vi "dump data from VIs.vi"(7 "vipb base":path, 8 "error in (no error)":errorcluster, 9 "palette sections":T1(array[cluster]), 10 "assets":path, 11 "docs folder":path) -> (0 "error out":errorcluster)   [LabVIEW 2020]
uses:
  <vilib>/JDP Science/JSONtext/LVClass Serializer/JSONtext LVClass Serializer.lvclass
  sphinx terminal direction.ctl
  sphinx terminal data.ctl
  sphinx item data.ctl
  <vilib>/Utility/Data Type/NI_Data Type.lvlib
  41f7d256-710a-436a-832c-a9b2a359d6cb.vi
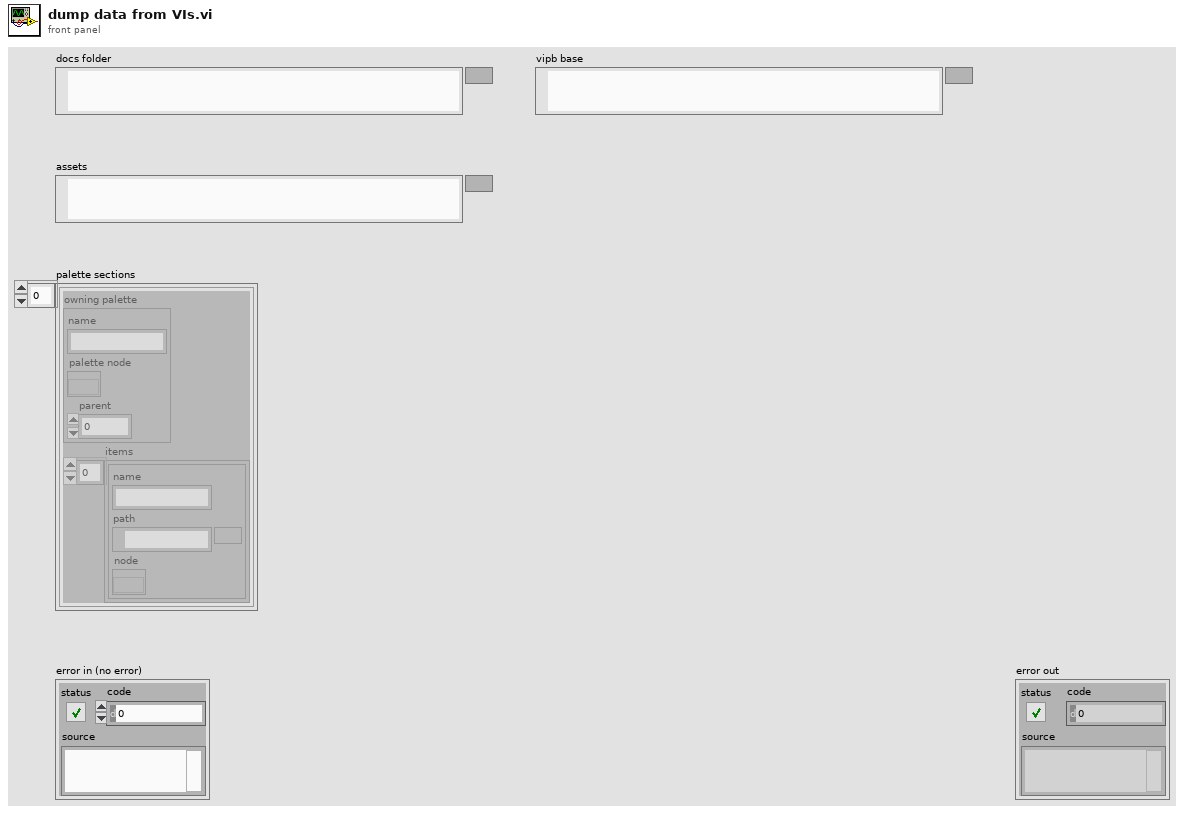
[diagram p1: front panel]
types:
  T1 = cluster{"owning palette":cluster{"name":string, "palette node":refnum<k20>, "parent":i32}, "items":cluster{"name":string, "path":path, "node":refnum<k20>}[]}[]
  T2 = typedef "sphinx item data.ctl" = cluster{"id":string, "kind":string, "path":path, "owner":string, "description":string, "icon":path, "terminals":T3[], "relative palette location":string, "connpane":path, "parent ID":string}
  T3 = typedef "sphinx terminal data.ctl" = cluster{"label":string, "direction":T4, "type":string, "type_id":string, "default":string, "description":string, "tip strip":string, "wiring rule":enum16{"Invalid Wire Rule", "Required", "Recommended", "Optional", "Dynamic Dispatch"}, "caption":string}
  T4 = typedef "sphinx terminal direction.ctl" = enum16{"input", "output"}
  T5 = enum16{"open", "replace", "create", "open or create", "replace or create", "replace or create with confirmation"}
  T6 = cluster{"name":string, "palette node":refnum<k20>, "parent":i32}
  T7 = cluster{"name":string, "path":path, "node":refnum<k20>}[]
  T8 = enum32{"invalid VI type", "Standard VI", "Control VI", "Global VI", "Polymorphic VI", "Configuration VI", "SubSystem", "Facade VI", "Method VI", "Statechart Diagram VI"}
  T9 = cluster{"VIPath":path, "Menu Name":string, "Selector Name":string}[]
  T10 = enum16{"Invalid Wire Rule", "Required", "Recommended", "Optional", "Dynamic Dispatch"}
  T11 = typedef "NI_Data Type.lvlib/Data Type.ctl" = enum8{"Invalid Type", "Void", "I8", "I16", "I32", "I64", "U8", "U16", "U32", "U64", "Single Float", "Double Float", "Extended Float", "Single Complex", "Double Complex", "Extended Complex", "Enum U8", "Enum U16", "Enum U32", "Enum U64", "Single Float With Unit", "Double Float With Unit", "Extended Float With Unit", "Single Complex with Unit", "Double Complex with Unit", "Extended Complex with Unit", "Boolean", "String", "Path", "Picture", "Tag", "Array", "Cluster", "Variant", "LV Variant", "Waveform", "Timestamp", "Digital Waveform", "Digital Data", "ExpressData", "Refnum", "External Data", "VI", "Poly VI", "LabVIEW Class Instance", "Fixed Point", "Set Collection", "Map Collection"}
  T12 = typedef "NI_Data Type.lvlib/Type Definition Info.ctl" = cluster{"Name":string, "Timestamp":u32}
  T13 = typedef "imagedata.ctl" = cluster{"image type":i32, "image depth":i32, "image":u8[], "mask":u8[], "colors":u32[], "Rectangle":cluster{"left":i16, "top":i16, "right":i16, "bottom":i16}}
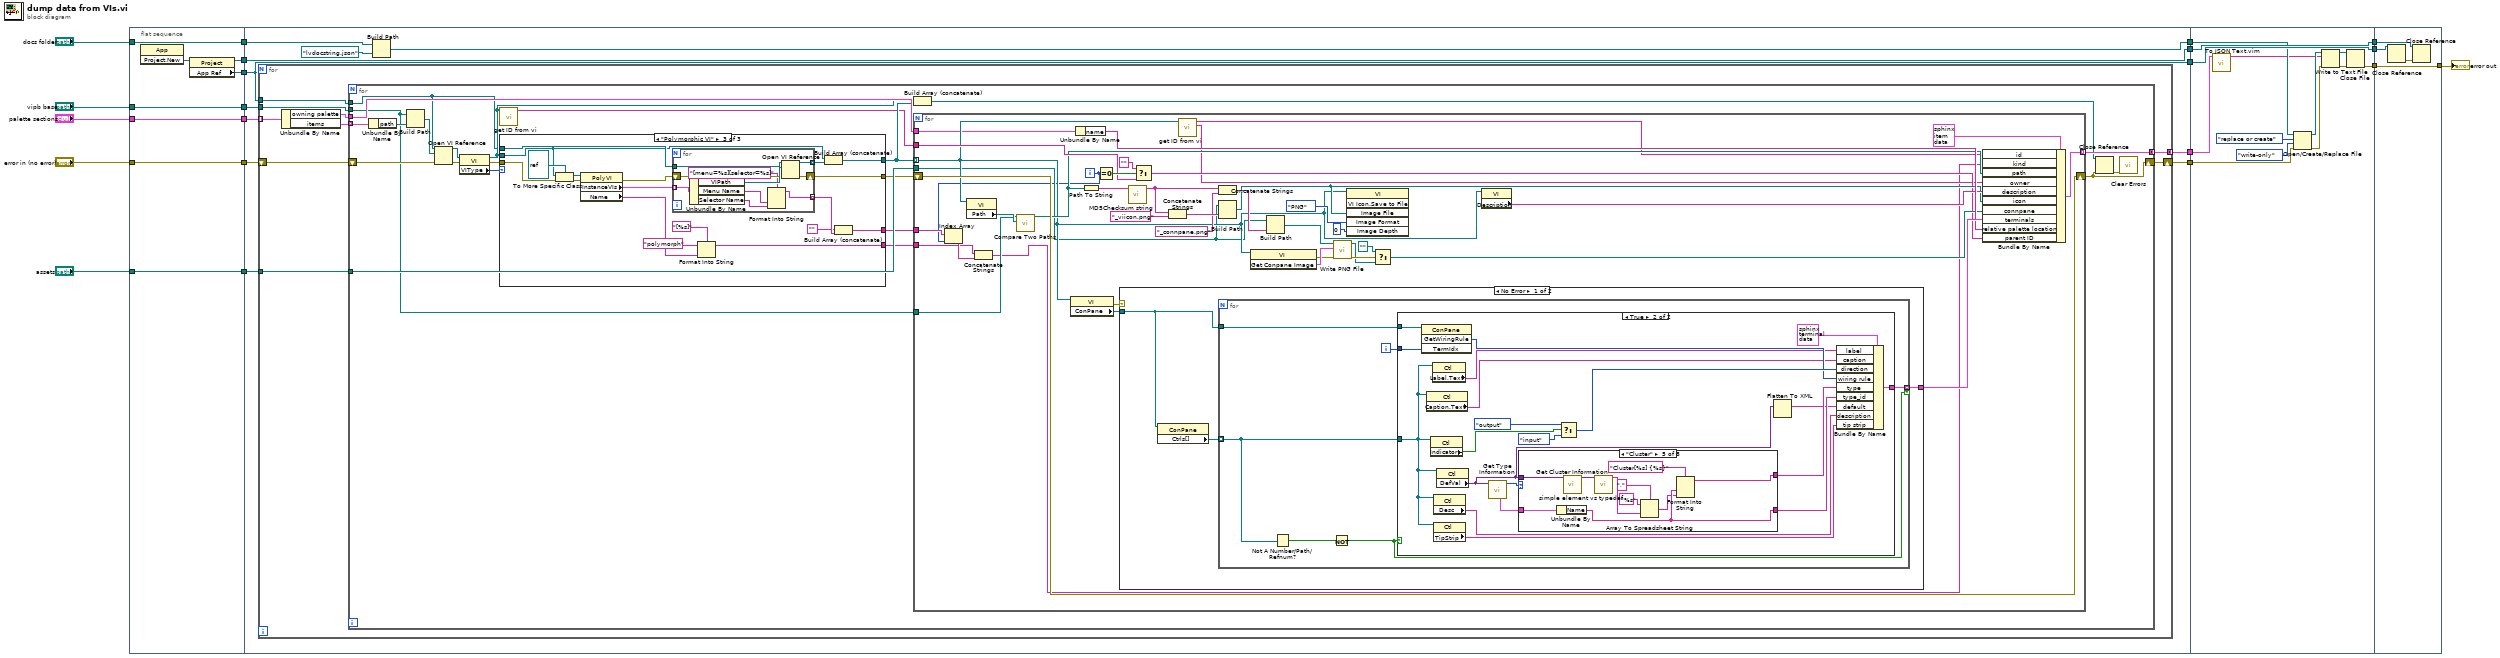
[diagram p0: block diagram]
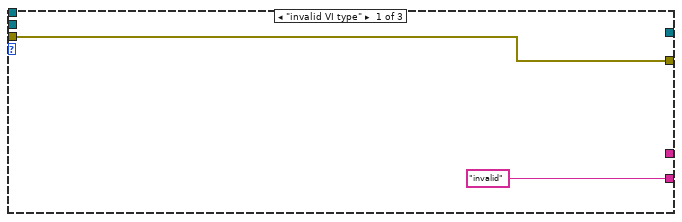
[diagram p2: hidden frame]
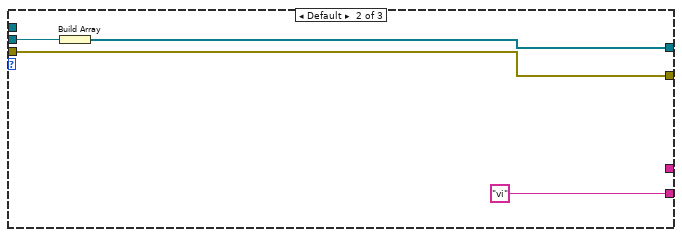
[diagram p3: hidden frame]
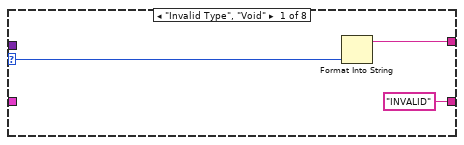
[diagram p5: hidden frame]
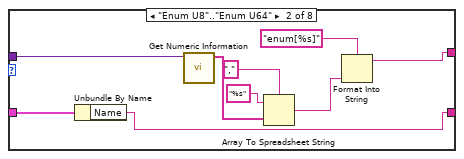
[diagram p6: hidden frame]
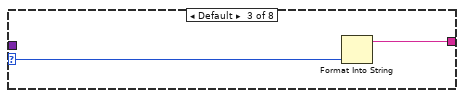
[diagram p7: hidden frame]
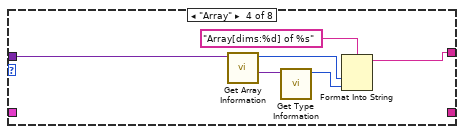
[diagram p8: hidden frame]
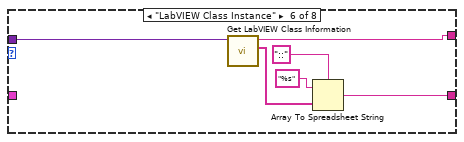
[diagram p9: hidden frame]
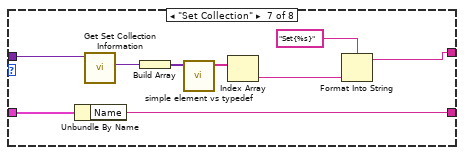
[diagram p10: hidden frame]
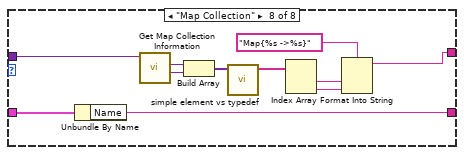
[diagram p11: hidden frame]
diagram:
  n1 = flat-sequence {
    tunnel: "palette sections" -> [w29]
    tunnel: [w29] -> w21
    tunnel: [w27] -> w20
    tunnel: [w26] -> w19
    tunnel: "error in (no error)" -> [w23]
    tunnel: "assets" -> [w25]
    tunnel: [w25] -> w18
    tunnel: [w24] -> w17
    tunnel: "docs folder" -> [w24]
    tunnel: [w23] -> w11
    tunnel: "vipb base" -> [w22]
    tunnel: [w22] -> w9
    tunnel: w21 -> [w40]
    tunnel: w20 -> [w39]
    tunnel: [w39] -> w8
    tunnel: [w38] -> w6
    tunnel: w19 -> [w38]
    tunnel: w18 -> [w37]
    tunnel: w17 -> [w36]
    tunnel: w11 -> [w34]
    tunnel: w9 -> [w33]
    tunnel: [w32] -> w3
    tunnel: [w31] -> w2
    tunnel: [w30] -> w1
    tunnel: w8 -> [w244]
    tunnel: [w244] -> w7
    tunnel: w6 -> [w243]
    tunnel: [w243] -> w5
    tunnel: [w234] -> w4
    tunnel: w3 -> [w238]
    tunnel: w2 -> [w235]
    tunnel: w1 -> [w233]
    tunnel: w7 -> [w247]
    tunnel: w5 -> [w246]
    tunnel: [w245] -> w16
    tunnel: w4 -> [w245]
    frame #0 {
      n2 = invoke class="App" method="Project.New"() -> ("Project:New"=w28:refnum<vi>)  [unwired: 3 in, 2 out]
      n3 = property class="Project"(reference=w28) -> (reference out=w27:refnum<vi>, "App Ref"=w26:refnum<vi>)  [unwired: 1 in, 1 out]
    }
    frame #1 {
      n4 = for {
        tunnel: w40 -> [w49] mode=indexing
        tunnel: w38 -> [w47]
        tunnel: [w45] -> w30 mode=concatenating
        tunnel: w37 -> [w44]
        shift-right: [w42] -> w32
        shift-left: w34 -> [w43]
        tunnel: w33 -> [w41]
        n5 = Unbundle By Name(w49) -> ("owning palette"=w46:T6, "items"=w48:T7)
        n6 = for {
          tunnel: w48 -> [w71] mode=indexing
          tunnel: w47 -> [w54]
          tunnel: w46 -> [w69]
          tunnel: [w68] -> w45 mode=concatenating
          tunnel: w44 -> [w67]
          shift-right: [w58] -> w42
          shift-left: w43 -> [w66]
          tunnel: w41 -> [w51]
          n7 = Unbundle By Name(w71) -> ("path"=w65:path)
          n8 = Build Path(base path=w51, name or relative path=w65) -> (appended path=w64:path)
          n9 = Open VI Reference(application reference (local)=w54, vi path=w64, error in (no error)=w66) -> (vi reference=w62:refnum<vi>, error out=w70:errorcluster)  [unwired: 3 in]
          n10 = property class="VI"(reference=w62, error in=w70) -> (reference out=w59:refnum<vi>, error out=w56:errorcluster, "VIType"=w60:T8)
          n11 = call "get ID from vi.vi"("VI in"=w59) -> ("VI ID"=w52:string)  [unwired: 9 in, 1 out]
          n12 = case shown="\"Polymorphic VI\"" w60 {
            tunnel: w59 -> [_ w77 w82]
            tunnel: [_ w76 w83] -> w61
            tunnel: [w73 w75 w89] -> w57
            tunnel: w56 -> [w73 w75 w95]
            tunnel: ["invalid" ("kind") "vi" ("kind") w81] -> w55
            tunnel: w54 -> [_ _ w91]
            tunnel: [_ _ w79] -> w50
            frame "invalid VI type" {
            }
            frame Default {
              n13 = Build Array(w77) -> (w76:refnum<vi>[])
            }
            frame "Polymorphic VI" {
              n14 = To More Specific Class(target class=refnum<vi> refnum, reference=w82, error in=w95) -> (specific class reference=w86:refnum<vi>, error out=w93:errorcluster)
              n15 = property class="PolyVI"(reference=w86, error in=w93) -> (error out=w90:errorcluster, "InstanceVIs"=w92:T9, "Name"=w85:string)  [unwired: 1 out]
              n16 = for {
                tunnel: w92 -> [w105] mode=indexing
                tunnel: w91 -> [w103]
                shift-right: [w101] -> w89
                shift-left: w90 -> [w102]
                tunnel: [w100] -> w88 mode=indexing
                tunnel: [w97] -> w80 mode=indexing
                n17 = Unbundle By Name(w105) -> ("VIPath"=w104:path, "Menu Name"=w99:string, "Selector Name"=w98:string)
                n18 = Format Into String(format string="[menu=%s][selector=%s]", w99, w98) -> (resulting string=w97:string)  [unwired: 2 in, 1 out]
                n19 = Open VI Reference(application reference (local)=w103, vi path=w104, error in (no error)=w102) -> (vi reference=w100:refnum<vi>, error out=w101:errorcluster)  [unwired: 3 in]
              }
              n20 = Format Into String(format string="[%s]", initial string="polymorph" ("kind"), w85) -> (resulting string=w81:string)  [unwired: 1 in, 1 out]
              n21 = Build Array (concatenate)(w82, w88) -> (w83:refnum<vi>[])
              n22 = Build Array (concatenate)("", w80) -> (w79:string[])
            }
          }
          n23 = Build Array (concatenate)(w59, w61) -> (w63:refnum<vi>[])
          n24 = for {
            tunnel: w69 -> [w112]
            tunnel: [w146] -> w68 mode=indexing
            tunnel: w67 -> [w111]
            shift-right: [w145] -> w58
            shift-left: w57 -> [w145]
            tunnel: w61 -> [w115] mode=indexing
            tunnel: w55 -> [w106]
            tunnel: w52 -> [w119]
            tunnel: w51 -> [w117]
            tunnel: w50 -> [w110]
            i -> [w109]
            n25 = Index Array(array=w110, index=w109) -> (element=w108:string)
            n26 = property class="VI"(reference=w115) -> ("Path"=w118:path)  [unwired: 1 in, 2 out]
            n27 = Concatenate Strings(w106, w108) -> (w107:string)
            n28 = call <vilib>:"Compare Two Paths.vi"("Path 2"=w118, "Path 1"=w117) -> ("Relative Path from 1 to 2"=w116:path)  [unwired: 6 in, 3 out]
            n29 = property class="VI"(reference=w115) -> (error out=w128:errorcluster, "ConPane"=w129:refnum<vi>)  [unwired: 1 in, 1 out]
            n30 = Unbundle By Name(w112) -> ("name"=w139:string)
            n31 = Path To String(path=w116) -> (string=w137:string)
            n32 = Equal To 0?(x=w109) -> (x = 0?=w122:bool)
            n33 = case shown="No Error" w128 {
              tunnel: [w148 _] -> w140
              tunnel: w129 -> [w147 _]
              frame No Error {
                n34 = property class="ConPane"(reference=w147) -> ("Ctrls[]"=w149:refnum<vi>[])  [unwired: 1 in, 2 out]
                n35 = for {
                  tunnel: w149 -> [w153] mode=indexing
                  tunnel: [w155] -> w148 mode=indexing if=w150
                  tunnel: w147 -> [w154]
                  i -> [w151]
                  n36 = Not A Number/Path/Refnum?(number/path/refnum=w153) -> (NaN/Path/Refnum?=w152:bool)
                  n37 = Not(x=w152) -> (.not. x?=w150:bool)
                  n38 = case shown="True" w150 {
                    tunnel: [_ w174] -> w155
                    tunnel: w154 -> [_ w167]
                    tunnel: w153 -> [_ w166]
                    tunnel: w151 -> [_ w165]
                    frame False {
                    }
                    frame True {
                      n39 = invoke class="ConPane" method="GetWiringRule"(reference=w167, "TermIdx"=w165) -> ("Get Wire Rule"=w164:T10)  [unwired: 2 in, 3 out]
                      n40 = property class="Ctl"(reference=w166) -> ("Caption.Text"=w157:string)  [unwired: 1 in, 2 out]
                      n41 = property class="Ctl"(reference=w166) -> ("Indicator"=w173:bool)  [unwired: 1 in, 2 out]
                      n42 = property class="Ctl"(reference=w166) -> ("Label.Text"=w156:string)  [unwired: 1 in, 2 out]
                      n43 = property class="Ctl"(reference=w166) -> ("Desc"=w168:string)  [unwired: 1 in, 2 out]
                      n44 = property class="Ctl"(reference=w166) -> ("TipStrip"=w169:string)  [unwired: 1 in, 2 out]
                      n45 = property class="Ctl"(reference=w166) -> ("DefVal"=w159:variant)  [unwired: 1 in, 2 out]
                      n46 = call <vilib>:"Get Type Information.vi"("variant"=w159) -> ("type"=w163:T11, "type definition info"=w161:T12)  [unwired: 6 in, 3 out]
                      n47 = case shown="\"Cluster\"" w163 {
                        selector: w163 -> [w176 _ w189 _ _ _ _ _]
                        tunnel: ["INVALID" w186 _ _ w204 w206 w213 w224] -> w162
                        tunnel: w161 -> [_ w187 _ _ w205 _ w214 w225]
                        tunnel: [w177 w180 w188 w190 w197 w210 w215 w226] -> w160
                        tunnel: w159 -> [_ w185 _ w195 w201 w211 w220 w231]
                        frame "Invalid Type", "Void" {
                          n48 = Format Into String(w176) -> (resulting string=w177:string)  [unwired: 3 in, 1 out]
                        }
                        frame "Enum U8".."Enum U64" {
                          n49 = Unbundle By Name(w187) -> ("Name"=w186:string)
                          n50 = call <vilib>:"Get Numeric Information.vi"("variant"=w185) -> ("enum names"=w184:string[])  [unwired: 7 in, 3 out]
                          n51 = Array To Spreadsheet String(delimiter (Tab)=",", array=w184, 3:"%s" ("format string")) -> (spreadsheet string=w183:string)
                          n52 = Format Into String(format string="enum[%s]", w183) -> (resulting string=w180:string)  [unwired: 2 in, 1 out]
                        }
                        frame Default {
                          n53 = Format Into String(w189) -> (resulting string=w188:string)  [unwired: 3 in, 1 out]
                        }
                        frame "Array" {
                          n54 = call <vilib>:"Get Array Information.vi"("variant"=w195) -> ("array element data type"=w192:variant, "number of dimensions"=w193:i32)  [unwired: 7 in, 2 out]
                          n55 = call <vilib>:"Get Type Information.vi"("variant"=w192) -> ("type"=w191:T11)  [unwired: 6 in, 4 out]
                          n56 = Format Into String(format string="Array[dims:%d] of %s", w193, w191) -> (resulting string=w190:string)  [unwired: 2 in, 1 out]
                        }
                        frame "Cluster" {
                          n57 = Unbundle By Name(w205) -> ("Name"=w204:string)
                          n58 = call <vilib>:"Get Cluster Information.vi"("variant"=w201) -> ("cluster elements"=w200:variant[])  [unwired: 9 in, 1 out]
                          n59 = call "simple element vs typedef.vi"("elements"=w200) -> ("simple identifiers"=w199:string[])  [unwired: 10 in]
                          n60 = Array To Spreadsheet String(delimiter (Tab)=",", array=w199, 3:"%s" ("format string")) -> (spreadsheet string=w202:string)
                          n61 = Format Into String(format string="Cluster[%s] {%s}", w204, w202) -> (resulting string=w197:string)  [unwired: 2 in, 1 out]
                        }
                        frame "LabVIEW Class Instance" {
                          n62 = call <vilib>:"Get LabVIEW Class Information.vi"("variant"=w211) -> ("qualified LabVIEW class name"=w207:string[], "LabVIEW class file name"=w210:string)  [unwired: 8 in, 1 out]
                          n63 = Array To Spreadsheet String(delimiter (Tab)="::", array=w207, 3:"%s" ("format string")) -> (spreadsheet string=w206:string)
                        }
                        frame "Set Collection" {
                          n64 = Unbundle By Name(w214) -> ("Name"=w213:string)
                          n65 = call <vilib>:"Get Set Collection Information.vi"("variant"=w220) -> ("element data type"=w219:variant)  [unwired: 9 in, 1 out]
                          n66 = Build Array(w219) -> (w218:variant[])
                          n67 = call "simple element vs typedef.vi"("elements"=w218) -> ("simple identifiers"=w217:string[])  [unwired: 10 in]
                          n68 = Index Array(array=w217) -> (element=w216:string)  [unwired: 1 in]
                          n69 = Format Into String(format string="Set{%s}", w216) -> (resulting string=w215:string)  [unwired: 2 in, 1 out]
                        }
                        frame "Map Collection" {
                          n70 = Unbundle By Name(w225) -> ("Name"=w224:string)
                          n71 = call <vilib>:"Get Map Collection Information.vi"("variant"=w231) -> ("value data type"=w222:variant, "key data type"=w230:variant)  [unwired: 8 in, 1 out]
                          n72 = Build Array(w230, w222) -> (w229:variant[])
                          n73 = call "simple element vs typedef.vi"("elements"=w229) -> ("simple identifiers"=w228:string[])  [unwired: 10 in]
                          n74 = Index Array(array=w228) -> (element #1=w227:string, element #2=w221:string)  [unwired: 2 in]
                          n75 = Format Into String(format string="Map{%s ->%s}", w227, w221) -> (resulting string=w226:string)  [unwired: 2 in, 1 out]
                        }
                      }
                      n76 = Select(t=sphinx_terminal_direction."output" ("direction"), s=w173, f=sphinx_terminal_direction."input" ("direction")) -> (s? t:f=w170:T4)
                      n77 = Flatten To XML(6:w159) -> (2:w158:string)
                      n78 = Bundle By Name(cluster=T3 {"label"="", "direction"=enum."input", "type"="", "type_id"="", "default"="", "description"="", "tip strip"="", "wiring rule"=enum."Invalid Wire Rule", "caption"=""} ("Cluster"), "label"=w156, "caption"=w157, "direction"=w170, "wiring rule"=w164, "type"=w160, "type_id"=w162, "default"=w158, "description"=w168, "tip strip"=w169) -> (w174:T3)
                    }
                  }
                }
              }
              frame Error {
              }
            }
            n79 = call "MD5Checksum string.vi"("Message String"=w137) -> ("MD5 message-digest"=w131:string)  [unwired: 10 in]
            n80 = Select(t="", s=w122, f=w119) -> (s? t:f=w120:string)
            n81 = Concatenate Strings(w131, "_viicon.png" ("string")) -> (w135:string)
            n82 = call "get ID from vi.vi"("VI in"=w115) -> ("owning library"=w113:string, "VI ID"=w114:string)  [unwired: 9 in]
            n83 = Concatenate Strings(w131, "_connpane.png" ("string")) -> (w134:string)
            n84 = Build Path(base path=w111, name or relative path=w135) -> (appended path=w130:path)
            n85 = invoke class="VI" method="Get Conpane Image"(reference=w115) -> (error out=w127:errorcluster, "Get Conpane Image"=w142:T13)  [unwired: 2 in, 1 out]
            n86 = Build Path(base path=w111, name or relative path=w134) -> (appended path=w132:path)
            n87 = call <vilib>:"Write PNG File.vi"("error in (no error)"=w127, "image data"=w142, "path to PNG file"=w132) -> ("error out"=w126:errorcluster, "path"=w125:path)  [unwired: 7 in]
            n88 = invoke class="VI" method="VI Icon.Save to File"(reference=w115, "Image File"=w130, "Image Format"=enum32{"PNG", "JPEG", "GIF", "BMP"}."PNG", "Image Depth"=0) -> ()  [unwired: 2 in, 6 out]
            n89 = Select(t=path "", s=w126, f=w125) -> (s? t:f=w124:path)
            n90 = property class="VI"(reference=w115) -> ("Description"=w138:string)  [unwired: 1 in, 2 out]
            n91 = Bundle By Name(cluster=T2 {"id"="", "kind"="", "path"=path "", "owner"="", "description"="", "icon"=path "", "terminals"=[], "relative palette location"="", "connpane"=path "", "parent ID"=""} ("item"), "id"=w114, "kind"=w107, "path"=w116, "owner"=w113, "description"=w138, "icon"=w130, "connpane"=w124, "terminals"=w140, "relative palette location"=w139, "parent ID"=w120) -> (w146:T2)
          }
          n92 = Close Reference(reference=w63, error in (no error)=w58) -> (error out=w53:errorcluster)
          n93 = call <vilib>:"Clear Errors.vi"("error in (no error)"=w53) -> ()  [unwired: 5 in, 2 out]
        }
      }
      n94 = Build Path(base path=w36, name or relative path=path "lvdocstring.json") -> (appended path=w31:path)
    }
    frame #2 {
      n95 = call "To JSON Text.vim"("Anything"=w233) -> ("<JSON>"=w232:string)  [unwired: 9 in, 1 out]
      n96 = Open/Create/Replace File(file path (use dialog)=w235, error in=w238, operation (0:open)=T5."replace or create", access (0:read/write)=enum16{"read/write", "read-only", "write-only"}."write-only") -> (refnum out=w239:refnum<file>, error out=w240:errorcluster)  [unwired: 2 in, 1 out]
      n97 = Write to Text File(file (use dialog)=w239, text=w232, error in=w240) -> (refnum out=w241:refnum<file>, error out=w242:errorcluster)  [unwired: 1 in, 1 out]
      n98 = Close File(refnum=w241, error in=w242) -> (error out=w234:errorcluster)  [unwired: 1 out]
    }
    frame #3 {
      n99 = Close Reference(reference=w246) -> (error out=w248:errorcluster)  [unwired: 1 in]
      n100 = Close Reference(reference=w247, error in (no error)=w248) -> ()  [unwired: 1 out]
    }
  }
  "error out" <- w16
